vi "Barcode Scanner.vi"(8 "error in (no error)":errorcluster, 11 "reference":refnum<vi>) -> (0 "error in (no error) 2":errorcluster, 3 "reference 2":refnum<vi>)   [LabVIEW 2015]
uses:
  Control Button/Exit.ctl
  Enqueue/Test seqSB.ctl
  Enqueue/Test selectionSB.ctl
panel:
  in  "Previous Button":T1
  in  "Barcode Scanner":T2
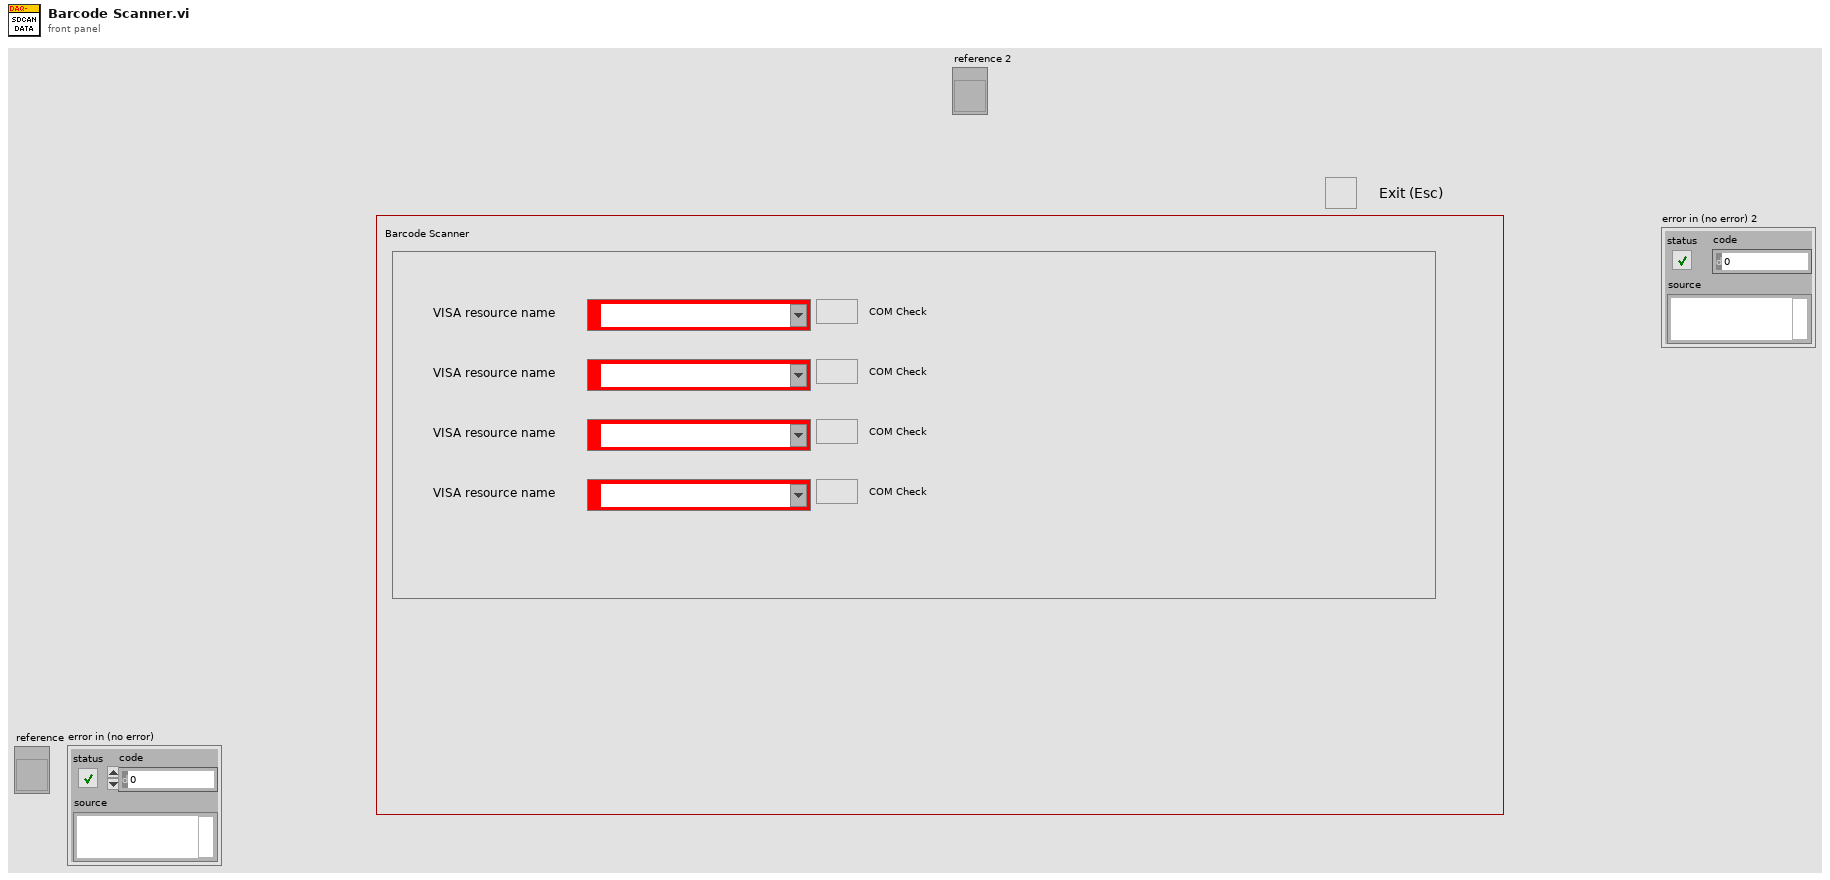
[diagram p1: front panel]
types:
  T1 = typedef "Exit.ctl" = bool
  T2 = cluster{"VISA resource name":refnum<visa-resource-name>, "ComPort":bool, "VISA resource name 2":refnum<visa-resource-name>, "ComPort 2":bool, "VISA resource name 3":refnum<visa-resource-name>, "ComPort 3":bool, "VISA resource name 4":refnum<visa-resource-name>, "ComPort 4":bool, "Scan Data":string, "Scan Data 2":string, "Scan Data 3":string, "Scan Data 4":string}
  T3 = typedef "Test seqSB.ctl" = enum16{"SBPoll Event", "SBinitialize", "SB Comport Check1", "SB Comport Check2", "SB Comport Check3", "SB Comport Check4", "SB Exit"}
  T4 = typedef "Test selectionSB.ctl" = enum16{"Init", "Enqueue ", "Enqueue N", "Enqueue in stack", "Enqueue in stack N", "Dequeue", "Dequeue N", "Flush", "Release Queue"}
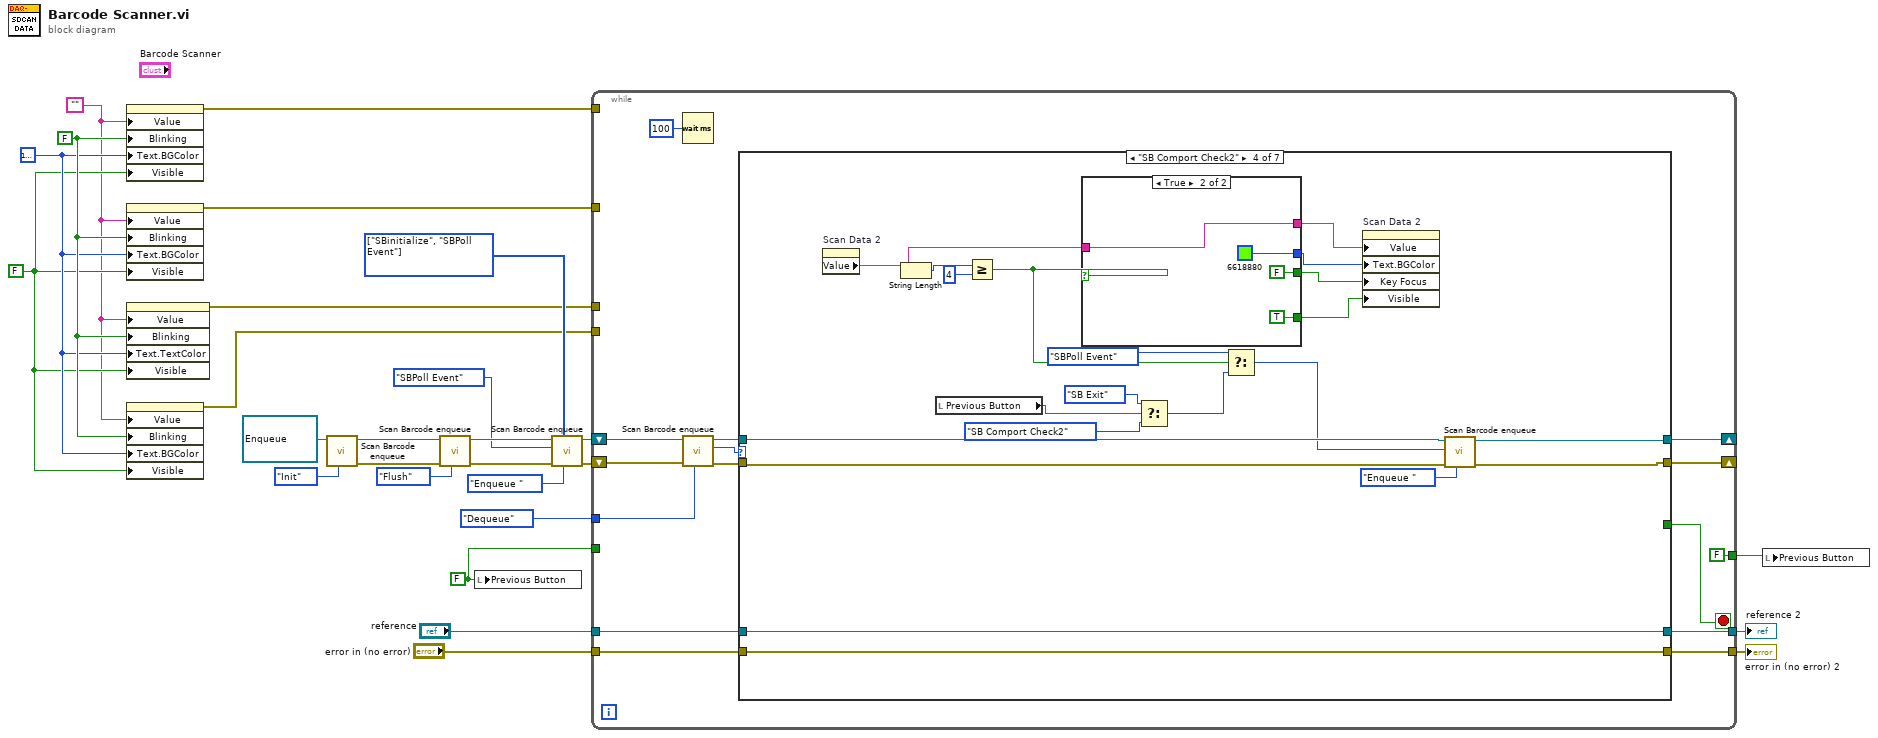
[diagram p0: block diagram]
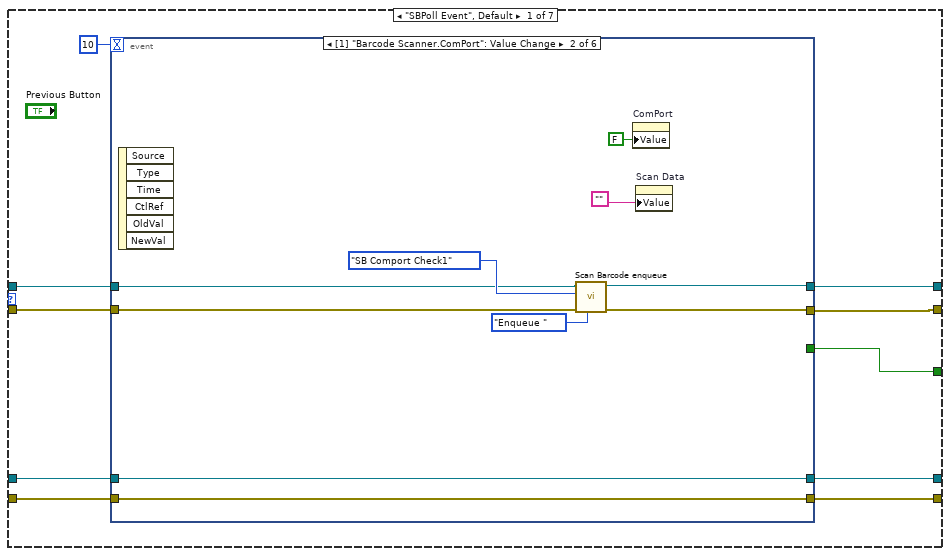
[diagram p2: hidden frame]
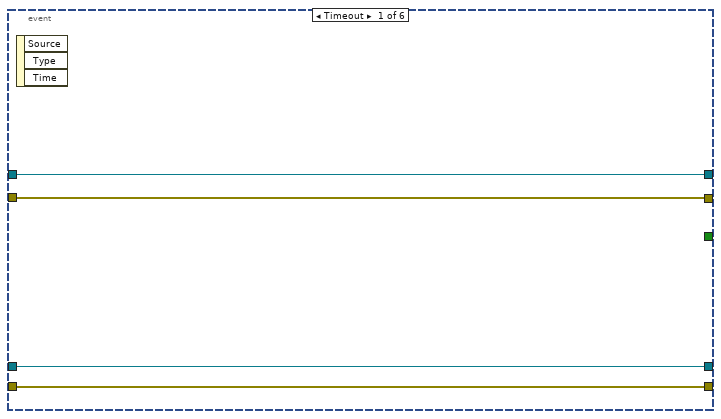
[diagram p3: hidden frame]
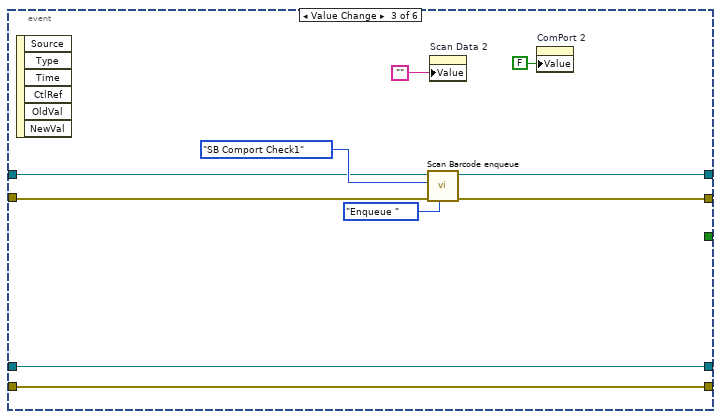
[diagram p4: hidden frame]
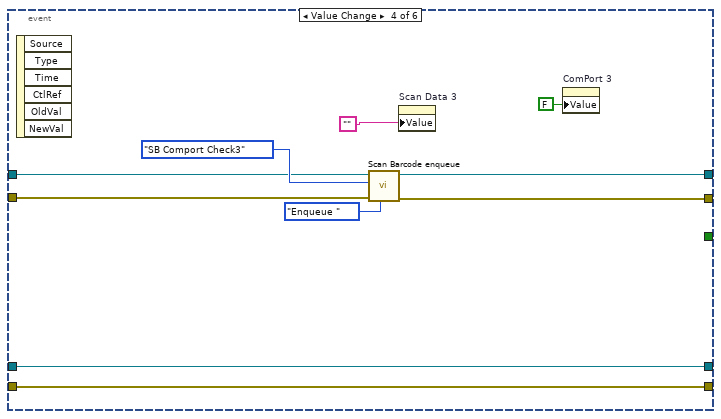
[diagram p5: hidden frame]
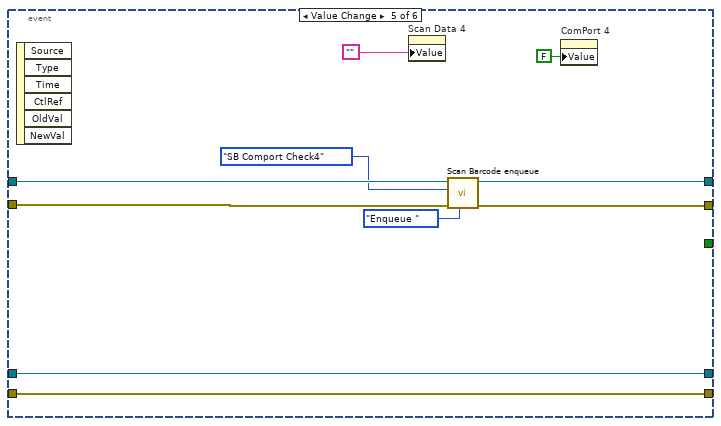
[diagram p6: hidden frame]
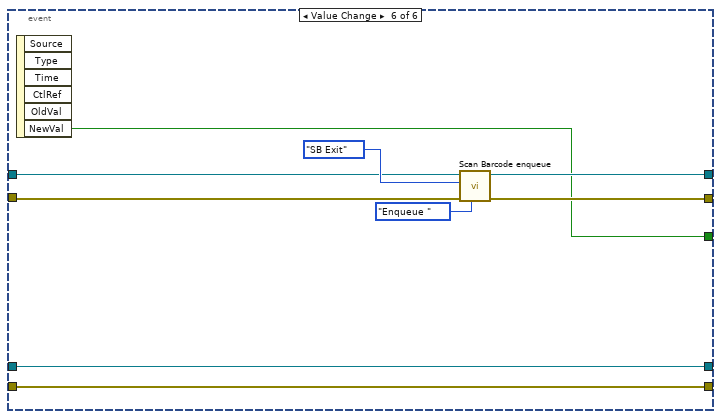
[diagram p7: hidden frame]
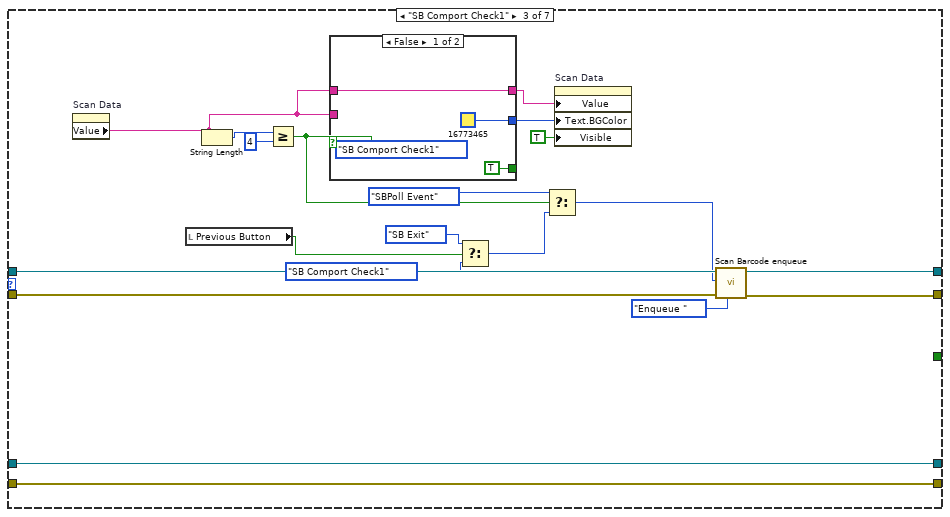
[diagram p9: hidden frame]
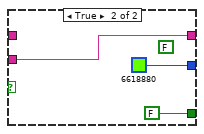
[diagram p10: hidden frame]
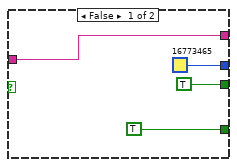
[diagram p11: hidden frame]
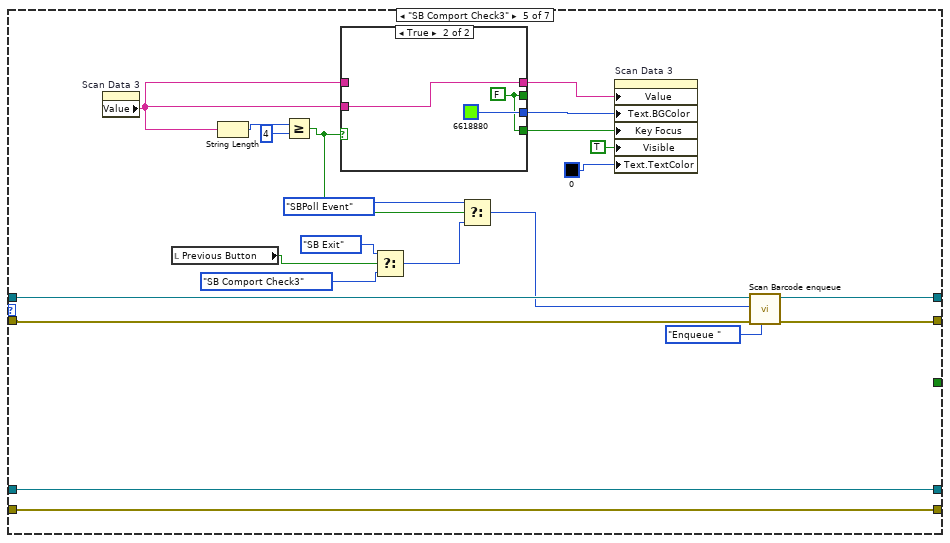
[diagram p12: hidden frame]
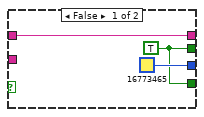
[diagram p13: hidden frame]
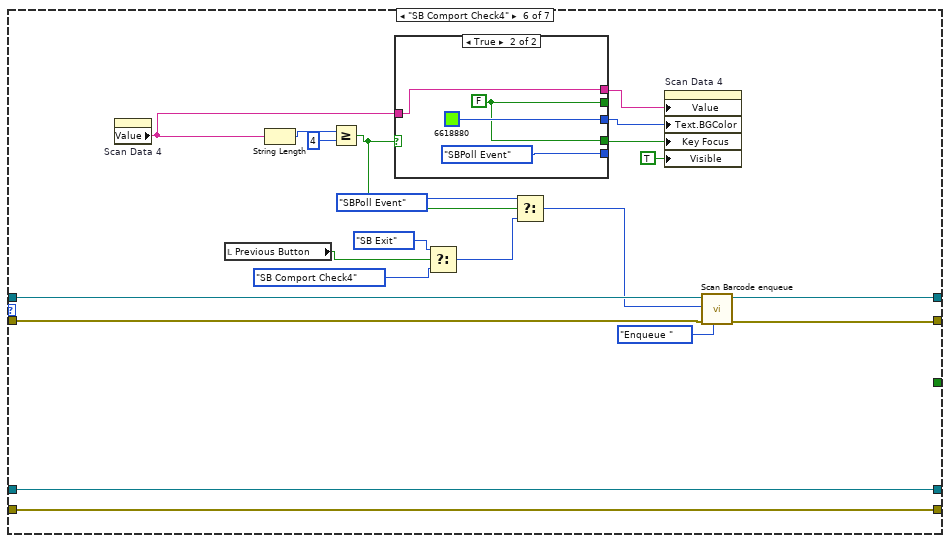
[diagram p14: hidden frame]
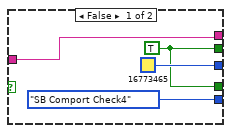
[diagram p15: hidden frame]
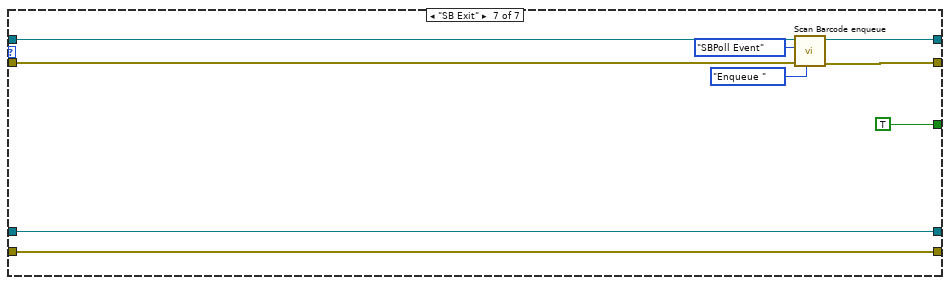
[diagram p16: hidden frame]
diagram:
  w6 = T1 FALSE ("Previous Button")
  w11 = ""
  w18 = T3[] [enum."SBinitialize", enum."SBPoll Event"] items=["SBPoll Event", "SBinitialize", "SB Comport Check1", "SB Comport Check2", "SB Comport Check3", "SB Comport Check4", "SB Exit"] ("Enqueue N")
  w24 = refnum<queue> refnum items=["SBPoll Event", "SBinitialize", "SB Comport Check1", "SB Comport Check2", "SB Comport Check3", "SB Comport Check4", "SB Exit"] ("queue in")
  w25 = FALSE ("Visible")
  w27 = FALSE ("Blinking")
  w26 = u32 16777225 ("Color Box")
  n1 = property on="Scan Data" class="Str"("Value"=w11, "Blinking"=w27, "Text.BGColor"=w26, "Visible"=w25) -> (error out=w10:errorcluster)  [unwired: 2 in, 1 out]
  n2 = property on="Scan Data 2" class="Str"("Value"=w11, "Blinking"=w27, "Text.BGColor"=w26, "Visible"=w25) -> (error out=w9:errorcluster)  [unwired: 2 in, 1 out]
  n3 = property on="Scan Data 3" class="Str"("Value"=w11, "Blinking"=w27, "Text.TextColor"=w26, "Visible"=w25) -> (error out=w8:errorcluster)  [unwired: 2 in, 1 out]
  n4 = property on="Scan Data 4" class="Str"("Value"=w11, "Blinking"=w27, "Text.BGColor"=w26, "Visible"=w25) -> (error out=w7:errorcluster)  [unwired: 2 in, 1 out]
  n5 = call "Scan Barcode enqueue.vi"("Enum Selection"=Test_selectionSB."Init", "queue in"=w24) -> ("error out"=w22:errorcluster, "queue Out"=w16:refnum<queue>)  [unwired: 6 in, 1 out]
  n6 = call "Scan Barcode enqueue.vi"("Enum Selection"=Test_selectionSB."Flush", "Error In"=w22, "queue in"=w16) -> ("error out"=w19:errorcluster, "queue Out"=w15:refnum<queue>)  [unwired: 5 in, 1 out]
  n7 = local write "Previous Button"(w6) -> ()
  n8 = call "Scan Barcode enqueue.vi"("Enum Selection"=Test_selectionSB."Enqueue ", "Enqueue N"=w18, "Error In"=w19, "Enqueue"=Test_seqSB."SBPoll Event", "queue in"=w15) -> ("error out"=w14:errorcluster, "queue Out"=w17:refnum<queue>)  [unwired: 3 in, 1 out]
  n9 = while {
    shift-right: [w42] -> _
    shift-left: w17 -> [w41]
    shift-right: [w38] -> _
    shift-left: w14 -> [w37]
    tunnel: Test_selectionSB."Dequeue" ("Enum Selection") -> [w35]
    tunnel: w10 -> [_]
    tunnel: w9 -> [_]
    tunnel: w8 -> [_]
    tunnel: w7 -> [_]
    tunnel: w6 -> [_]
    tunnel: [T1 FALSE ("Previous Button")] -> w5
    tunnel: "reference" -> [w31]
    tunnel: "error in (no error)" -> [w30]
    tunnel: [w29] -> w2
    tunnel: [w28] -> w1
    stop <- w33 stop-if-true
    n10 = Wait (ms)(milliseconds to wait=u32 100) -> ()  [unwired: 1 out]
    n11 = call "Scan Barcode enqueue.vi"("Enum Selection"=w35, "Error In"=w37, "queue in"=w41) -> ("error out"=w39:errorcluster, "D-enqueue"=w36:T3, "queue Out"=w40:refnum<queue>)  [unwired: 5 in]
    n12 = case shown="\"SB Comport Check2\"" w36 {
      tunnel: w40 -> [w51 w109 w125 w153 w183 w211 w227]
      tunnel: [w49 w109 w123 w155 w185 w213 w229] -> w42
      tunnel: w39 -> [w50 w108 w124 w152 w182 w210 w226]
      tunnel: [w48 w108 w122 w154 w184 w212 w228] -> w38
      tunnel: [w47 _ _ _ _ _ TRUE] -> w33
      tunnel: w31 -> [w46 w106 w110 w136 w165 w193 w222]
      tunnel: w30 -> [w45 w107 w111 w137 w166 w194 w223]
      tunnel: [w44 w106 w110 w136 w165 w193 w222] -> w29
      tunnel: [w43 w107 w111 w137 w166 w194 w223] -> w28
      frame "SBPoll Event", Default {
        n13 = event shown="[1] \"Barcode Scanner.ComPort\": Value Change" {
          selector: _ -> [_ _ _ _ _ _]
          dyn-events: _ -> [_ _ _ _ _ _]
          timeout: 10 -> [_ _ _ _ _ _]
          tunnel: w51 -> [w56 w62 w71 w84 w95 w103]
          tunnel: w50 -> [w55 w64 w72 w82 w94 w102]
          tunnel: [w56 w61 w74 w83 w93 w100] -> w49
          tunnel: [w55 w63 w73 w81 w92 w101] -> w48
          tunnel: [_ _ _ _ _ w99] -> w47
          tunnel: w46 -> [w54 w58 w68 w78 w88 w98]
          tunnel: w45 -> [w53 w57 w67 w77 w87 w97]
          tunnel: [w54 w58 w68 w78 w88 w98] -> w44
          tunnel: [w53 w57 w67 w77 w87 w97] -> w43
          event Timeout {
            n14 = event-data() -> ()  [unwired: 1 in, 3 out]
          }
          event "Barcode Scanner.ComPort": Value Change {
            n15 = event-data() -> ()  [unwired: 1 in, 6 out]
            n16 = call "Scan Barcode enqueue.vi"("Enum Selection"=Test_selectionSB."Enqueue ", "Error In"=w64, "Enqueue"=Test_seqSB."SB Comport Check1", "queue in"=w62) -> ("error out"=w63:errorcluster, "queue Out"=w61:refnum<queue>)  [unwired: 4 in, 1 out]
            n17 = property on="ComPort" class="Bool (strict)"("Value"=FALSE) -> ()  [unwired: 2 in, 2 out]
            n18 = property on="Scan Data" class="Str"("Value"="") -> ()  [unwired: 2 in, 2 out]
          }
          event "Barcode Scanner.ComPort 2": Value Change {
            n19 = event-data() -> ()  [unwired: 1 in, 6 out]
            n20 = call "Scan Barcode enqueue.vi"("Enum Selection"=Test_selectionSB."Enqueue ", "Error In"=w72, "Enqueue"=Test_seqSB."SB Comport Check1", "queue in"=w71) -> ("error out"=w73:errorcluster, "queue Out"=w74:refnum<queue>)  [unwired: 4 in, 1 out]
            n21 = property on="Scan Data 2" class="Str"("Value"="") -> ()  [unwired: 2 in, 2 out]
            n22 = property on="ComPort 2" class="Bool (strict)"("Value"=FALSE) -> ()  [unwired: 2 in, 2 out]
          }
          event "Barcode Scanner.ComPort 3": Value Change {
            n23 = event-data() -> ()  [unwired: 1 in, 6 out]
            n24 = call "Scan Barcode enqueue.vi"("Enum Selection"=Test_selectionSB."Enqueue ", "Error In"=w82, "Enqueue"=Test_seqSB."SB Comport Check3", "queue in"=w84) -> ("error out"=w81:errorcluster, "queue Out"=w83:refnum<queue>)  [unwired: 4 in, 1 out]
            n25 = property on="Scan Data 3" class="Str"("Value"="") -> ()  [unwired: 2 in, 2 out]
            n26 = property on="ComPort 3" class="Bool (strict)"("Value"=FALSE) -> ()  [unwired: 2 in, 2 out]
          }
          event "Barcode Scanner.ComPort 4": Value Change {
            n27 = event-data() -> ()  [unwired: 1 in, 6 out]
            n28 = property on="Scan Data 4" class="Str"("Value"="") -> ()  [unwired: 2 in, 2 out]
            n29 = call "Scan Barcode enqueue.vi"("Enum Selection"=Test_selectionSB."Enqueue ", "Error In"=w94, "Enqueue"=Test_seqSB."SB Comport Check4", "queue in"=w95) -> ("error out"=w92:errorcluster, "queue Out"=w93:refnum<queue>)  [unwired: 4 in, 1 out]
            n30 = property on="ComPort 4" class="Bool (strict)"("Value"=FALSE) -> ()  [unwired: 2 in, 2 out]
          }
          event Value Change {
            n31 = event-data() -> ("NewVal"=w99:T1)  [unwired: 1 in, 5 out]
            n32 = call "Scan Barcode enqueue.vi"("Enum Selection"=Test_selectionSB."Enqueue ", "Error In"=w102, "Enqueue"=Test_seqSB."SB Exit", "queue in"=w103) -> ("error out"=w101:errorcluster, "queue Out"=w100:refnum<queue>)  [unwired: 4 in, 1 out]
          }
        }
      }
      frame "SBinitialize" {
      }
      frame "SB Comport Check1" {
        n33 = property on="Scan Data" class="Str"() -> ("Value"=w119:string)  [unwired: 2 in, 2 out]
        n34 = local read "Previous Button"() -> (w116:T1)
        n35 = String Length(string=w119) -> (length=w129:i32)
        n36 = Greater Or Equal?(x=w129, y=4) -> (x >= y?=w115:bool)
        n37 = case shown="False" w115 {
          tunnel: w119 -> [w132 _]
          tunnel: [w132 w135] -> w120
          tunnel: w119 -> [_ w135]
          tunnel: [u32 16773465 ("Color Box") u32 6618880 ("Color Box")] -> w127
          tunnel: [TRUE ("Key Focus") FALSE ("Key Focus")] -> _
          frame False {
            (unwired) Test_seqSB."SB Comport Check1" ("Enqueue")
          }
          frame True {
            (unwired) FALSE
          }
        }
        n38 = Select(t=Test_seqSB."SB Exit" ("Enqueue"), s=w116, f=Test_seqSB."SB Comport Check1" ("Enqueue")) -> (s? t:f=w112:T3)
        n39 = Select(t=Test_seqSB."SBPoll Event" ("Enqueue"), s=w115, f=w112) -> (s? t:f=w117:T3)
        n40 = property on="Scan Data" class="Str"("Value"=w120, "Text.BGColor"=w127, "Visible"=TRUE) -> ()  [unwired: 2 in, 2 out]
        n41 = call "Scan Barcode enqueue.vi"("Enum Selection"=Test_selectionSB."Enqueue ", "Error In"=w124, "Enqueue"=w117, "queue in"=w125) -> ("error out"=w122:errorcluster, "queue Out"=w123:refnum<queue>)  [unwired: 4 in, 1 out]
      }
      frame "SB Comport Check2" {
        n42 = property on="Scan Data 2" class="Str"() -> ("Value"=w146:string)  [unwired: 2 in, 2 out]
        n43 = String Length(string=w146) -> (length=w151:i32)
        n44 = local read "Previous Button"() -> (w144:T1)
        n45 = Greater Or Equal?(x=w151, y=4) -> (x >= y?=w139:bool)
        n46 = case shown="True" w139 {
          tunnel: [w157 w164] -> w145
          tunnel: w146 -> [w157 w164]
          tunnel: [u32 16773465 ("Color Box") u32 6618880 ("Color Box")] -> w149
          tunnel: [TRUE ("Visible") TRUE ("Visible")] -> w148
          tunnel: [TRUE FALSE] -> w147
          frame False {
          }
          frame True {
          }
        }
        n47 = Select(t=Test_seqSB."SB Exit" ("Enqueue"), s=w144, f=Test_seqSB."SB Comport Check2" ("Enqueue")) -> (s? t:f=w140:T3)
        n48 = Select(t=Test_seqSB."SBPoll Event" ("Enqueue"), s=w139, f=w140) -> (s? t:f=w138:T3)
        n49 = property on="Scan Data 2" class="Str"("Value"=w145, "Text.BGColor"=w149, "Key Focus"=w147, "Visible"=w148) -> ()  [unwired: 2 in, 2 out]
        n50 = call "Scan Barcode enqueue.vi"("Enum Selection"=Test_selectionSB."Enqueue ", "Error In"=w152, "Enqueue"=w138, "queue in"=w153) -> ("error out"=w154:errorcluster, "queue Out"=w155:refnum<queue>)  [unwired: 4 in, 1 out]
      }
      frame "SB Comport Check3" {
        n51 = property on="Scan Data 3" class="Str"() -> ("Value"=w175:string)  [unwired: 2 in, 2 out]
        n52 = local read "Previous Button"() -> (w173:T1)
        n53 = String Length(string=w175) -> (length=w181:i32)
        n54 = Greater Or Equal?(x=w181, y=4) -> (x >= y?=w168:bool)
        n55 = case shown="True" w168 {
          tunnel: w175 -> [w189 _]
          tunnel: [w189 w192] -> w176
          tunnel: w175 -> [_ w192]
          tunnel: [u32 16773465 ("Color Box") u32 6618880 ("Color Box")] -> w179
          tunnel: [w187 w190] -> _
          tunnel: [w187 w190] -> w178
          frame False {
            w187 = TRUE
          }
          frame True {
            w190 = FALSE
          }
        }
        n56 = Select(t=Test_seqSB."SB Exit" ("Enqueue"), s=w173, f=Test_seqSB."SB Comport Check3" ("Enqueue")) -> (s? t:f=w169:T3)
        n57 = Select(t=Test_seqSB."SBPoll Event" ("Enqueue"), s=w168, f=w169) -> (s? t:f=w167:T3)
        n58 = property on="Scan Data 3" class="Str"("Value"=w176, "Text.BGColor"=w179, "Key Focus"=w178, "Visible"=TRUE, "Text.TextColor"=u32 0 ("Color Box")) -> ()  [unwired: 2 in, 2 out]
        n59 = call "Scan Barcode enqueue.vi"("Enum Selection"=Test_selectionSB."Enqueue ", "Error In"=w182, "Enqueue"=w167, "queue in"=w183) -> ("error out"=w184:errorcluster, "queue Out"=w185:refnum<queue>)  [unwired: 4 in, 1 out]
      }
      frame "SB Comport Check4" {
        n60 = property on="Scan Data 4" class="Str"() -> ("Value"=w203:string)  [unwired: 2 in, 2 out]
        n61 = local read "Previous Button"() -> (w201:T1)
        n62 = String Length(string=w203) -> (length=w209:i32)
        n63 = Greater Or Equal?(x=w209, y=4) -> (x >= y?=w196:bool)
        n64 = case shown="True" w196 {
          tunnel: [w214 w218] -> w202
          tunnel: w203 -> [w214 w218]
          tunnel: [u32 16773465 ("Color Box") u32 6618880 ("Color Box")] -> w207
          tunnel: [w216 w220] -> _
          tunnel: [w216 w220] -> w206
          tunnel: [Test_seqSB."SB Comport Check4" ("Enqueue") Test_seqSB."SBPoll Event" ("Enqueue")] -> _
          frame False {
            w216 = TRUE
          }
          frame True {
            w220 = FALSE
          }
        }
        n65 = Select(t=Test_seqSB."SB Exit" ("Enqueue"), s=w201, f=Test_seqSB."SB Comport Check4" ("Enqueue")) -> (s? t:f=w197:T3)
        n66 = Select(t=Test_seqSB."SBPoll Event" ("Enqueue"), s=w196, f=w197) -> (s? t:f=w195:T3)
        n67 = property on="Scan Data 4" class="Str"("Value"=w202, "Text.BGColor"=w207, "Key Focus"=w206, "Visible"=TRUE) -> ()  [unwired: 2 in, 2 out]
        n68 = call "Scan Barcode enqueue.vi"("Enum Selection"=Test_selectionSB."Enqueue ", "Error In"=w210, "Enqueue"=w195, "queue in"=w211) -> ("error out"=w212:errorcluster, "queue Out"=w213:refnum<queue>)  [unwired: 4 in, 1 out]
      }
      frame "SB Exit" {
        n69 = call "Scan Barcode enqueue.vi"("Enum Selection"=Test_selectionSB."Enqueue ", "Error In"=w226, "Enqueue"=Test_seqSB."SBPoll Event", "queue in"=w227) -> ("error out"=w228:errorcluster, "queue Out"=w229:refnum<queue>)  [unwired: 4 in, 1 out]
      }
    }
  }
  "reference 2" <- w2
  "error in (no error) 2" <- w1
  n70 = local write "Previous Button"(w5) -> ()
